vi "Stop Core.vi"(10 "final error code":i32, 11 "Ex Nested in":refnum<class "gController.lvclass">) -> (3 "Ex Nested out":refnum<class "gController.lvclass">)   [LabVIEW 2016, in "Controller.lvlib" / "gController.lvclass"]
doc: "(<B>Filename</B>: Actor Framework.lvlib:Actor.lvclass:Stop Core.vi)\n\nDefines what the actor does before it stops. Use the <B>final error code</B> input to determine whether the actor shut down in response to an error.\n\nBy default, this method does nothing. A descendant class may override it to define behavior, such as shutting down any processes the actor initiated in its override of the Actor Core method."
uses:
  gController.lvclass
  gController.lvclass/gController.ctl
  Data/SOAP Data.lvclass/SOAP Data.ctl
  Session/Raw FPGA/FPGA Session.lvclass
  C:/Program Files (x86)/National Instruments/LabVIEW 2016/vi.lib/MSR Consulting, LLC/General Reuse/Session APIs/_Session Fwk/Session - Root.lvclass
  Data/Read message_data.vi
  <vilib>/MSR Consulting, LLC/General Reuse/SuperActor/SuperActor.lvclass
  <vilib>/MSR Consulting, LLC/General Reuse/Session APIs/_Session Fwk/Session - Root.lvclass
  Data/SOAP Data.lvclass
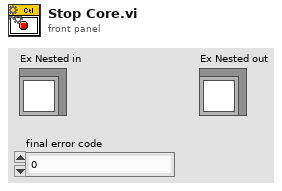
[diagram p1: front panel]
types:
  T1 = typedef "Session - Root.lvclass/Session Handle.ctl" = refnum<data-value>
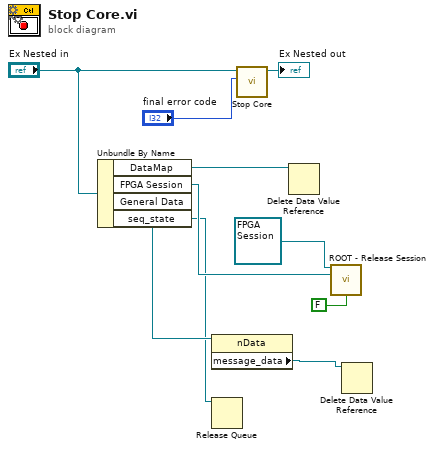
[diagram p0: block diagram]
diagram:
  n1 = Unbundle By Name("Ex Nested in") -> ("DataMap"=w7:refnum<data-value>, "FPGA Session"=w6:T1, "General Data"=w3:refnum<class "SOAP Data.lvclass">, "seq_state"=w1:refnum<queue>)
  n2 = property class="nData"(reference=w3) -> ("message_data"=w2:refnum<data-value>)  [unwired: 1 in, 2 out]
  n3 = Release Queue(queue=w1) -> ()  [unwired: 2 in, 3 out]
  n4 = call-parent "Stop Core.vi"("final error code"="final error code", "Ex Nested in"="Ex Nested in") -> ("Ex Nested out"=→"Ex Nested out":refnum<class "gController.lvclass">)  [unwired: 9 in]
  n5 = Delete Data Value Reference(data value reference=w7) -> ()  [unwired: 1 in, 2 out]
  n6 = call <vilib>:"ROOT - Release Session.vi"("OBJ - Session in"=refnum<class "FPGA Session.lvclass"> refnum ("FPGA Session"), "Session Handle in"=w6, "force destroy? (F)"=FALSE) -> ()  [unwired: 11 in, 2 out]
  n7 = Delete Data Value Reference(data value reference=w2) -> ()  [unwired: 1 in, 2 out]
